vi "CSV Second Checker.vi"() -> ()   [LabVIEW 2021]
uses:
  <vilib>/Utility/file.llb/Read Delimited Spreadsheet (string).vi
panel:
  out "Error Data Points":string[](array[string])
  out "ERROR DETECTED":bool
  out "String":string
  out "Loop Iteration":i32
  out "Seconds Between Points":i16
  out "Extracted Seconds":i16
  out "match + rest of string":string
  out "substring before match":string
  out "delimited string":string
  out "first subarray":string[](array[string])
  out "array w/ subset deleted":string[](array[string])
  out "deleted portion":string
  out "subarray":string[](array[string])
  out "size(s)":i32
  out "all rows":string[][](array[string])
  out "error out":errorcluster
  in  "File Path":path
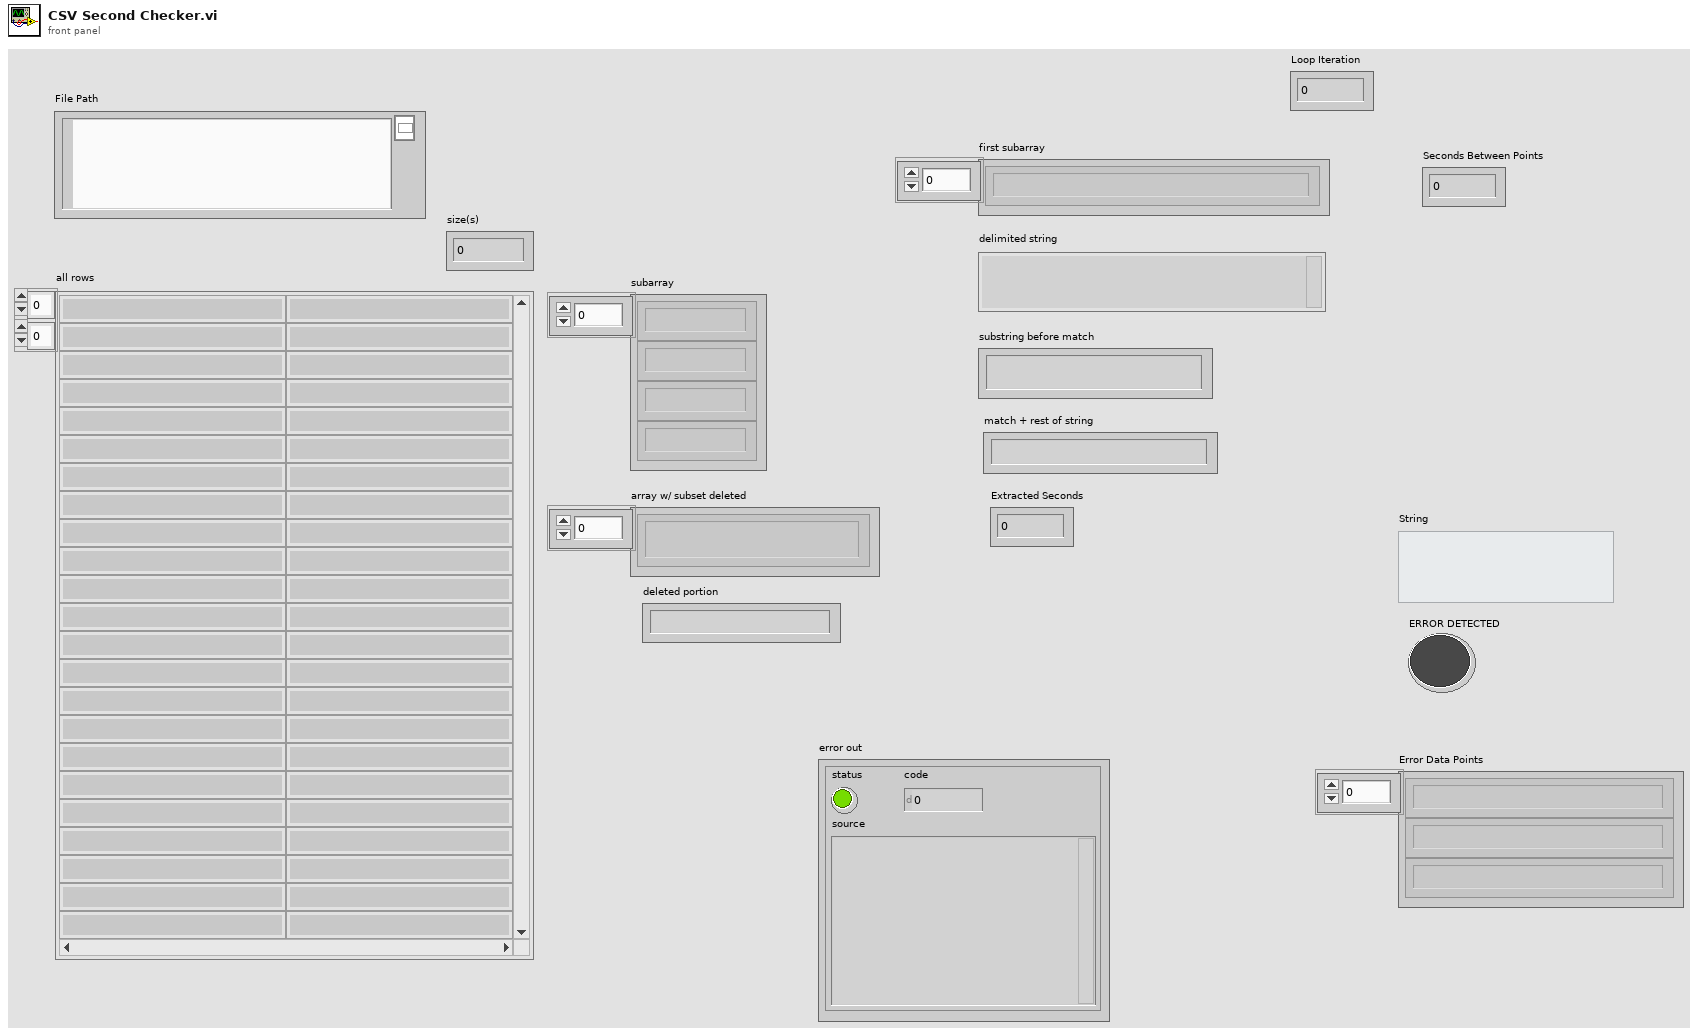
[diagram p1: front panel]
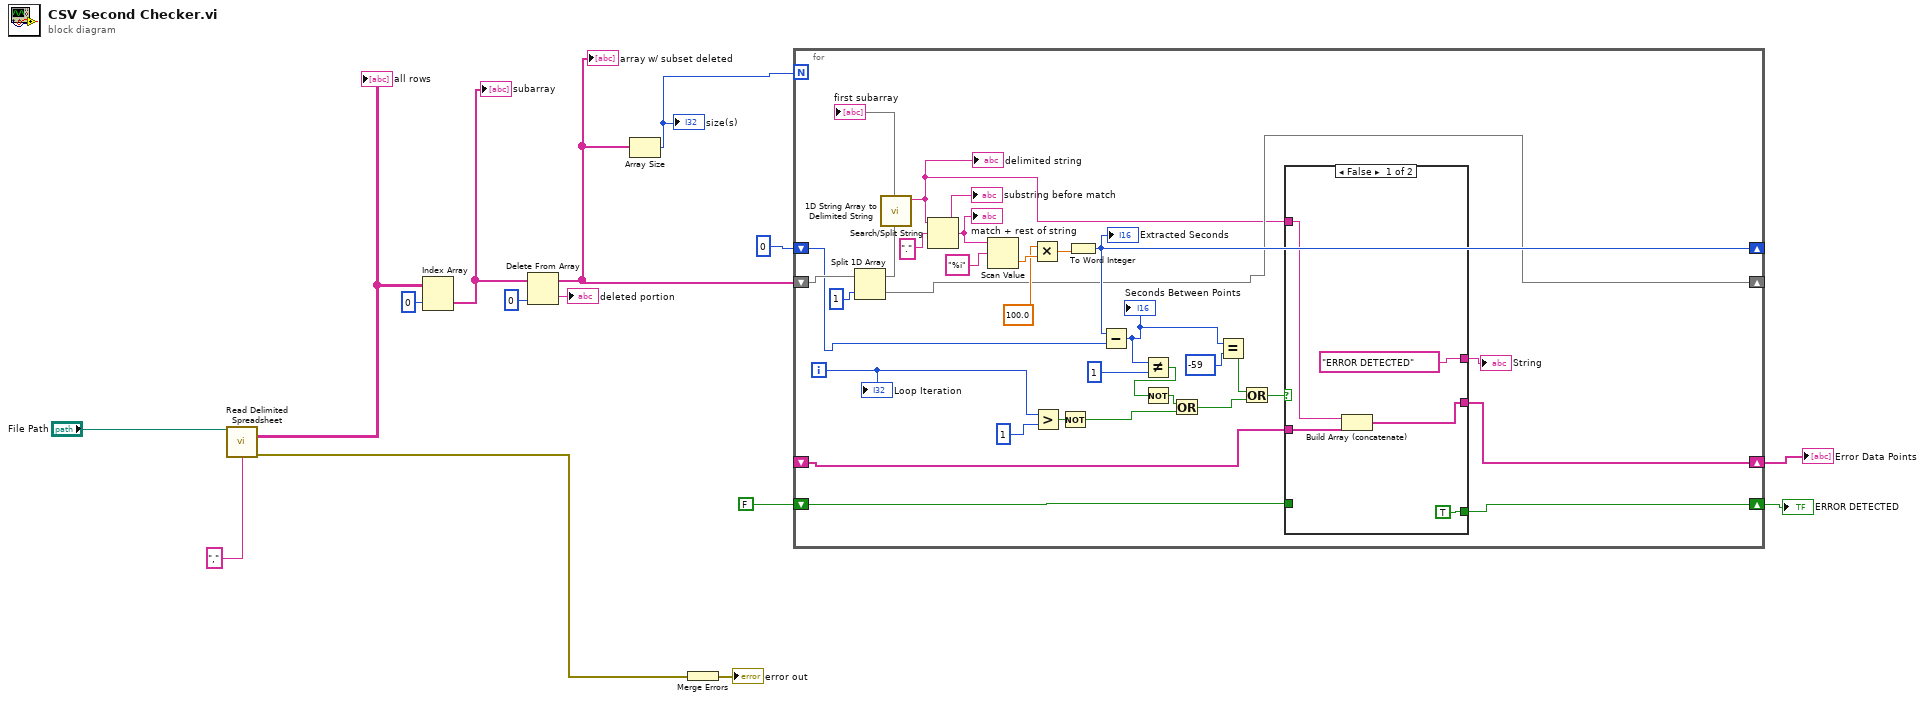
[diagram p0: block diagram]
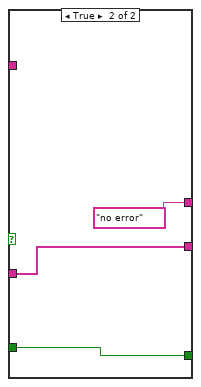
[diagram p2: hidden frame]
diagram:
  n1 = call-poly <vilib>:"Read Delimited Spreadsheet.vi"("file path (dialog if empty)"="File Path", "delimiter (\\t)"="," ("delimiter (\\t)")) -> ("all rows"=w11:string[][], "error out"=w13:errorcluster)  [unwired: 8 in, 4 out]
  "all rows" <- w11
  n2 = Index Array "Index Array"(array=w11, index (col)=0 ("disabled index (col)")) -> (element=w9:string[])  [unwired: 1 in]
  "subarray" <- w9
  n3 = Delete From Array(array=w9, index=0) -> (deleted portion=→"deleted portion":string, array with subset deleted=w6:string[])  [unwired: 1 in]
  "array w/ subset deleted" <- w6
  n4 = Array Size(array=w6) -> (size(s)=w4:i32)
  "size(s)" <- w4
  n5 = Merge Errors(w13) -> (→"error out":errorcluster)
  n6 = for {
    N: w4 -> [_]
    shift-right: [w17] -> _
    shift-left: w6 -> [w46]
    shift-right: [w36] -> _
    shift-left: i16 0 -> [w35]
    shift-right: [w26] -> w1
    shift-left: _ -> [w25]
    shift-right: [w22] -> w2
    shift-left: FALSE -> [w21]
    i -> [w27]
    n7 = Split 1D Array(array=w46, index=1) -> (first subarray=w44:string[], second subarray=w17:string[])
    "first subarray" <- w44
    n8 = call <vilib>:"1D String Array to Delimited String.vi"("string array"=w44) -> ("delimited string"=w16:string)  [unwired: 10 in]
    "delimited string" <- w16
    n9 = Search/Split String(string=w16, search string/char (-)="." ("regular expression")) -> (substring before match=→"substring before match":string, match + rest of string=w41:string)  [unwired: 1 in, 1 out]
    "match + rest of string" <- w41
    n10 = Scan Value(string=w41, format string="%i") -> (value=w39:dbl)  [unwired: 1 in, 1 out]
    n11 = Multiply(x=100.0, y=w39) -> (x*y=w37:dbl)
    n12 = Greater?(x=w27, y=1) -> (0:w34:bool)
    n13 = Not(x=w34) -> (.not. x?=w32:bool)
    n14 = To Word Integer(number=w37) -> (16bit integer=w36:i16)
    "Extracted Seconds" <- w36
    n15 = Subtract(x=w36, y=w35) -> (x-y=w20:i16)
    "Seconds Between Points" <- w20
    n16 = Not Equal?(x=w20, y=i16 1) -> (x != y?=w18:bool)
    n17 = Not(x=w18) -> (.not. x?=w24:bool)
    n18 = Or(x=w24, y=w32) -> (x .or. y?=w29:bool)
    n19 = Equal?(x=w20, y=-59) -> (x = y?=w30:bool)
    n20 = Or(x=w30, y=w29) -> (x .or. y?=w28:bool)
    n21 = case shown="False" w28 {
      tunnel: [w47 w54] -> w26
      tunnel: w25 -> [w48 w54]
      tunnel: ["ERROR DETECTED" ("String") "no error" ("String")] -> w23
      tunnel: [TRUE w52] -> w22
      tunnel: w21 -> [_ w52]
      tunnel: w16 -> [w49 _]
      frame False {
        n22 = Build Array (concatenate)(w49, w48) -> (w47:string[])
      }
      frame True {
      }
    }
    "String" <- w23
    "Loop Iteration" <- w27
  }
  "ERROR DETECTED" <- w2
  "Error Data Points" <- w1
